vi "Generate DAQ Waveform.vi"(7 "DAQ Config Data":T1, 8 "error in (no error)":errorcluster, 9 "Channel Data":dbl[](array[numeric]), 11 "Phase Array In":dbl[](array[numeric])) -> (0 "error out":errorcluster, 2 "Waveform Array":waveform(dbl)[](array[waveform]), 3 "Phase Array Out out":dbl[](array[numeric]))   [LabVIEW 2020, in "Waveform Analog Output Engine.lvlib"]
doc: "Create an array of waveforms based on the channel settings from the VeriStand engine"
uses:
  Waveform Analog Output Engine.lvlib
  DAQ Config Data.ctl
  <vilib>/measure/NI_MABase.lvlib
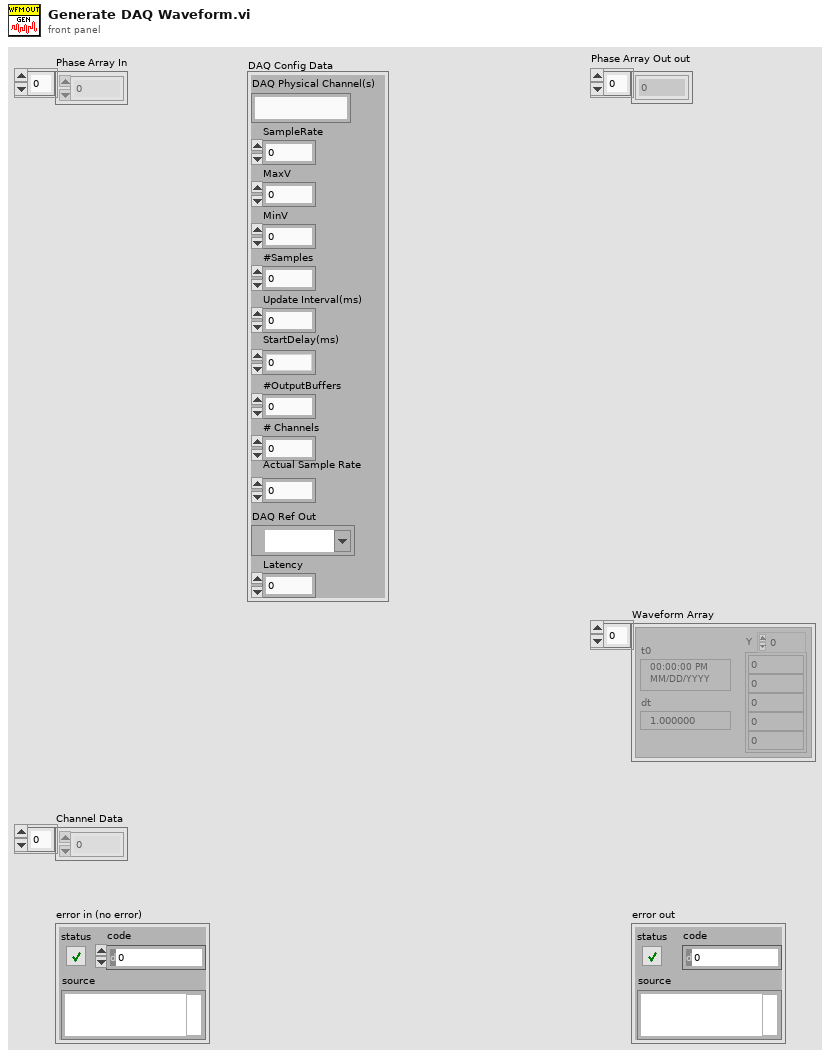
[diagram p1: front panel]
types:
  T1 = typedef "Waveform Analog Output Engine.lvlib/DAQ Config Data.ctl" = cluster{"DAQ Physical Channel(s)":string, "SampleRate":dbl, "MaxV":dbl, "MinV":dbl, "#Samples":dbl, "Update Interval(ms)":u32, "StartDelay(ms)":dbl, "#OutputBuffers":dbl, "# Channels":i32, "Actual Sample Rate":dbl, "DAQ Ref Out":refnum<k21>, "Latency":dbl}
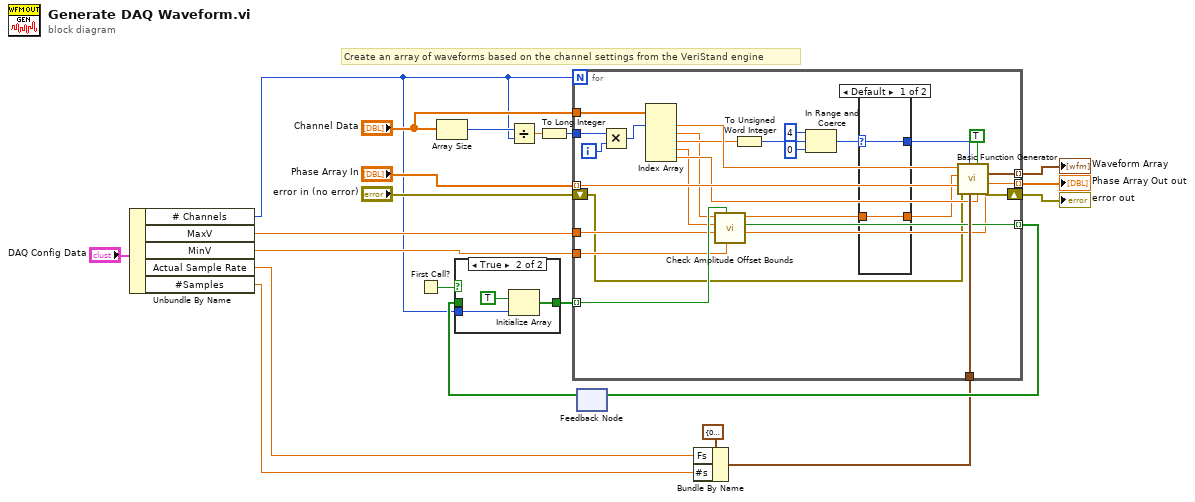
[diagram p0: block diagram]
diagram:
  # "Create an array of waveforms based on the channel settings from the VeriStand engine"
  n1 = Unbundle By Name("DAQ Config Data") -> ("# Channels"=w1:i32, "MaxV"=w9:dbl, "MinV"=w8:dbl, "Actual Sample Rate"=w4:dbl, "#Samples"=w3:dbl)
  n2 = First Call?() -> (First Call?: T/F=w12:bool)
  n3 = Array Size(array="Channel Data") -> (size(s)=w19:i32)
  n4 = Divide(x=w19, y=w1) -> (x/y=w20:dbl)
  n5 = To Long Integer(number=w20) -> (32bit integer=w21:i32)
  n6 = feedback #1() -> (w6:bool[])  [unwired: 1 in]
  n7 = case shown="True" w12 {
    tunnel: w1 -> [_ w25]
    tunnel: [w22 w23] -> w11
    tunnel: w6 -> [w22 _]
    frame False {
    }
    frame True {
      n8 = Initialize Array(TRUE, w25) -> (w23:bool[])
    }
  }
  n9 = Bundle By Name(cluster=cluster{"Fs":dbl, "#s":dbl} {"Fs"=0.0, "#s"=0.0} ("sampling info"), "Fs"=w4, "#s"=w3) -> (w2:cluster{"Fs":dbl, "#s":dbl})
  n10 = for {
    N: w1 -> [_]
    tunnel: w2 -> [w53]
    tunnel: [w52] -> w13 mode=indexing
    tunnel: [w51] -> w15 mode=indexing
    tunnel: "Phase Array In" -> [w50] mode=indexing
    shift-right: [w49] -> w17
    shift-left: "error in (no error)" -> [w30]
    tunnel: "Channel Data" -> [w48]
    tunnel: w21 -> [w43]
    tunnel: w11 -> [w41] mode=indexing
    tunnel: w9 -> [w38]
    tunnel: w8 -> [w39]
    tunnel: [w40] -> w7 mode=indexing
    i -> [w47]
    n11 = Multiply(x=w43, y=w47) -> (x*y=w46:i32)
    n12 = Index Array(array=w48, index #1=w46) -> (element #1=w45:dbl, element #2=w34:dbl, element #3=w44:dbl, element #4=w36:dbl, element #5=w37:dbl)  [unwired: 4 in]
    n13 = call "Check Amplitude Offset Bounds.vi"("MinV"=w39, "Last Iter In Bounds?"=w41, "MaxV"=w38, "Offset"=w36, "Amplitude"=w34) -> ("Coerced Offset"=w35:dbl, "Values In Bounds?"=w40:bool, "Coerced Amplitude"=w33:dbl)  [unwired: 4 in]
    n14 = To Unsigned Word Integer(number=w44) -> (unsigned 16bit integer=w27:u16)
    n15 = In Range and Coerce(upper limit=u16 4, x=w27, lower limit=u16 0) -> (coerced(x)=w26:u16)  [unwired: 1 out]
    n16 = case shown="Default" w26 {
      selector: w26 -> [w54 _]
      tunnel: w33 -> [w55 _]
      tunnel: [w55 _] -> w32
      tunnel: [w54 _] -> w31
      frame Default {
      }
      frame 4 {
        # "DC"
      }
    }
    n17 = call <vilib>:"Basic Function Generator.vi"("offset"=w35, "square wave duty cycle (%)"=w37, "reset signal"=TRUE, "sampling info"=w53, "signal type"=w31, "error in (no error)"=w30, "phase"=w50, "amplitude"=w32, "frequency"=w45) -> ("error out"=w49:errorcluster, "phase out"=w51:dbl, "signal out"=w52:waveform(dbl))
  }
  "error out" <- w17
  "Phase Array Out out" <- w15
  "Waveform Array" <- w13
  n18 = feedback-in #1(w7) -> ()
